vi "PS3 Controller.vi"(8 "error in (no error)":errorcluster, 11 "device ID":refnum<k1>) -> (0 "error out":errorcluster, 2 "Buttons control":T1, 3 "Control cluster":T2 {"Roll" scale=-1.0..1.0; "Pitch" scale=-1.0..1.0; "Vertical Speed" scale=-1.0..1.0; "Yaw Speed" scale=-1.0..1.0})   [LabVIEW 2014]
uses:
  <vilib>/Utility/inputDevices.llb/joystickAcquire.vi
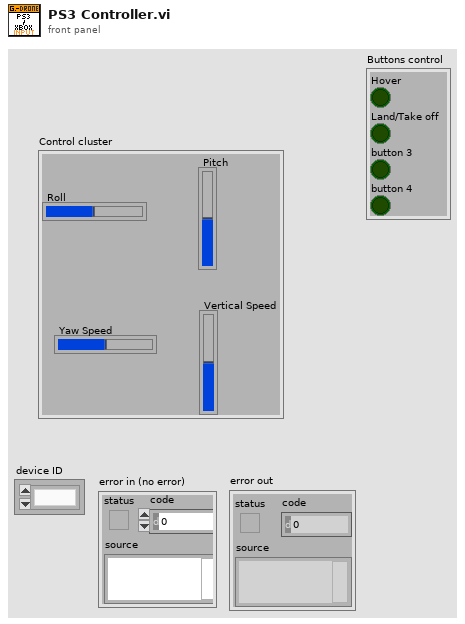
[diagram p1: front panel]
types:
  T1 = cluster{"Hover":bool, "Land/Take off":bool, "button 3":bool, "button 4":bool}
  T2 = cluster{"Roll":dbl, "Pitch":dbl, "Vertical Speed":dbl, "Yaw Speed":dbl}
  T3 = cluster{"X axis":i32, "Y axis":i32, "Z axis":i32, "X axis rotation":i32, "Y axis rotation":i32, "Z axis rotation":i32, "U axis":i32, "V axis":i32}
  T4 = cluster{"button 1":bool, "button 2":bool, "button 3":bool, "button 4":bool, "button 5":bool, "button 6":bool, "button 7":bool, "button 8":bool, "button 9":bool, "button 10":bool, "button 11":bool, "button 12":bool, "button 13":bool, "button 14":bool, "button 15":bool, "button 16":bool, "button 17":bool, "button 18":bool, "button 19":bool, "button 20":bool, "button 21":bool, "button 22":bool, "button 23":bool, "button 24":bool, "button 25":bool, "button 26":bool, "button 27":bool, "button 28":bool, "button 29":bool, "button 30":bool, "button 31":bool, "button 32":bool}
  T5 = cluster{"X axis":dbl, "Y axis":dbl, "Z axis":dbl, "X axis rotation":dbl, "Y axis rotation":dbl, "Z axis rotation":dbl, "U axis":dbl, "V axis":dbl}
  T6 = cluster{"button 1":bool, "button 2":bool, "button 3":bool, "button 4":bool}
  T7 = cluster{"X axis":dbl, "Y axis":dbl, "Z axis":dbl, "X axis rotation":dbl}
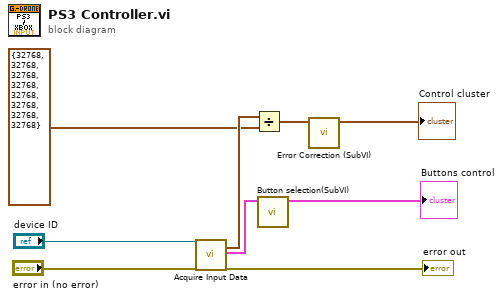
[diagram p0: block diagram]
diagram:
  n1 = call-poly <vilib>:"Acquire Input Data.vi"("device ID"="device ID", "error in (no error)"="error in (no error)") -> ("axis info"=w3:T3, "button info"=w6:T4, "error out"=→"error out":errorcluster)  [unwired: 13 in, 2 out]
  n2 = Divide(x=w3, y=T3 {"X axis"=32768, "Y axis"=32768, "Z axis"=32768, "X axis rotation"=32768, "Y axis rotation"=32768, "Z axis rotation"=32768, "U axis"=32768, "V axis"=32768}) -> (x/y=w4:T5)
  n3 = call "Button selection(SubVI).vi"("button info"=w6) -> ("Cluster"=→"Buttons control":T6)  [unwired: 10 in]
  n4 = call "Error Correction (SubVI).vi"("Cluster"=w4) -> ("cluster"=→"Control cluster":T7)  [unwired: 10 in]
